vi "RestartDevice.vi"(9 "SysCfgRestartRequest":T3, 11 "service":refnum<class "IcmMessageService.lvclass">) -> (2 "Header":T1, 3 "data string":string)   [LabVIEW 2016]
uses:
  <vilib>/addons/InsightCM/MessageBus/MessageService/IcmMessageService.lvclass
  <vilib>/addons/InsightCM/MessageBus/MessageLibrary/SysCfgDeployer/controls/SysCfgRestartRequestBody.ctl
  <vilib>/addons/InsightCM/MessageBus/Base/controls/KeyValuePair.ctl
  <vilib>/addons/InsightCM/MessageBus/Base/controls/MessageHeader.ctl
panel:
  in  "error in (no error)":errorcluster
  out "error out":errorcluster
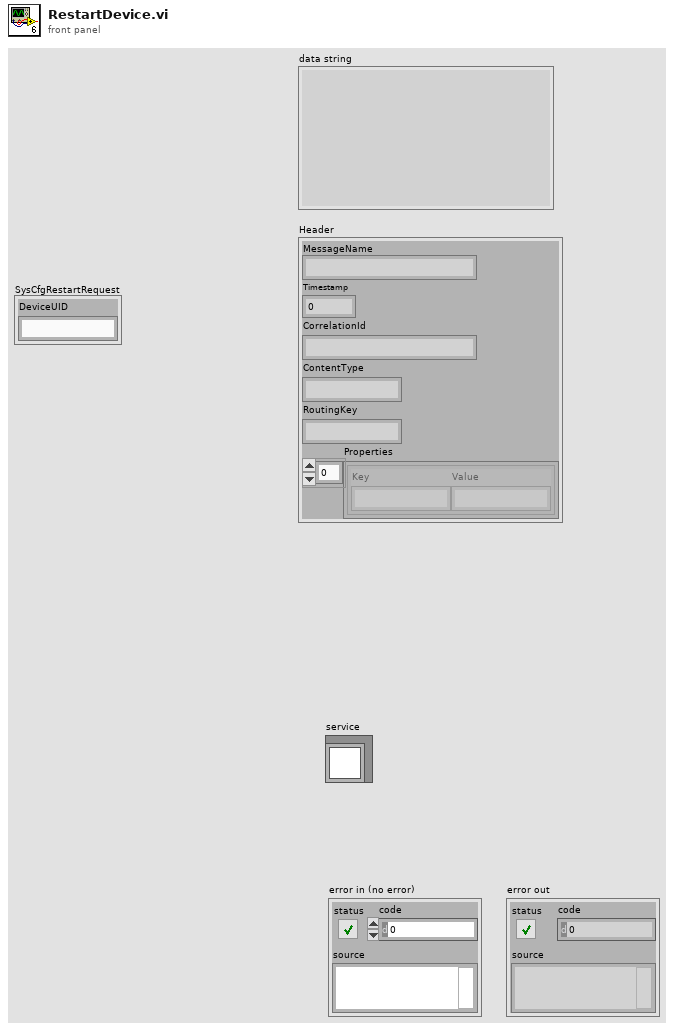
[diagram p1: front panel]
types:
  T1 = typedef "MessageHeader.ctl" = cluster{"MessageName":string, "Timestamp":i64, "CorrelationId":string, "ContentType":string, "RoutingKey":string, "Properties":T2[]}
  T2 = typedef "KeyValuePair.ctl" = cluster{"Key":string, "Value":string}
  T3 = typedef "SysCfgRestartRequestBody.ctl" = cluster{"DeviceUID":string}
  T4 = typedef "Message.ctl" = cluster{"Header":T1, "Body":u8[]}
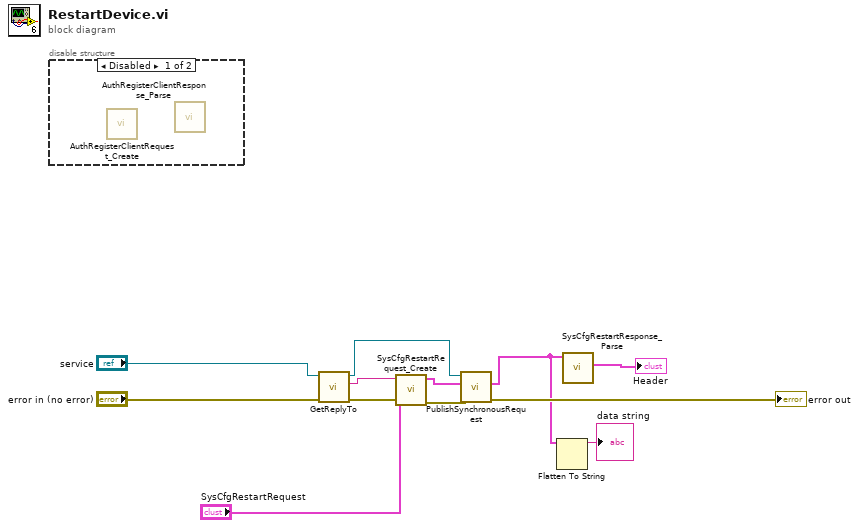
[diagram p0: block diagram]
diagram:
  n1 = disable-structure shown="Disabled" {
    frame Disabled {
      n2 = call <vilib>:"AuthRegisterClientRequest_Create.vi"() -> ()  [unwired: 10 in, 2 out]
      n3 = call <vilib>:"AuthRegisterClientResponse_Parse.vi"() -> ()  [unwired: 9 in, 3 out]
    }
    frame Enabled {
    }
  }
  n4 = call <vilib>:"GetReplyTo.vi"("error in (no error)"="error in (no error)", "service in"="service") -> ("error out"=w6:errorcluster, "reply to"=w7:string, "service out"=w10:refnum<class "IcmMessageService.lvclass">)  [unwired: 7 in]
  n5 = call <vilib>:"SysCfgRestartRequest_Create.vi"("error in (no error)"=w6, "SysCfgRestartRequest"="SysCfgRestartRequest", "ReplyTo"=w7) -> ("error out"=w5:errorcluster, "Message"=w4:T4)  [unwired: 7 in]
  n6 = call <vilib>:"PublishSynchronousRequest.vi"("error in (no error)"=w5, "request"=w4, "service in"=w10) -> ("error out"=→"error out":errorcluster, "response"=w2:T4)  [unwired: 6 in, 1 out]
  n7 = Flatten To String(anything=w2) -> (data string=→"data string":string)  [unwired: 3 in, 2 out]
  n8 = call <vilib>:"SysCfgRestartResponse_Parse.vi"("Message"=w2) -> ("Header"=→"Header":T1)  [unwired: 8 in, 2 out]
